vi "SPI读写.vi"(1 "DELAY":dbl, 3 "error in (no error)":errorcluster caption="错误输入（无错误）", 4 "从芯片读数据":string="spi r 0x04 0x0001", 5 "往芯片写数据":string="spi w 0x04 0x0001 0x01", 6 "VISA resource name":refnum<visa-resource-name>="COM3") -> (0 "error out":errorcluster, 2 "read buffer":string="spi read data is : 0xFF.")   [LabVIEW 2015]
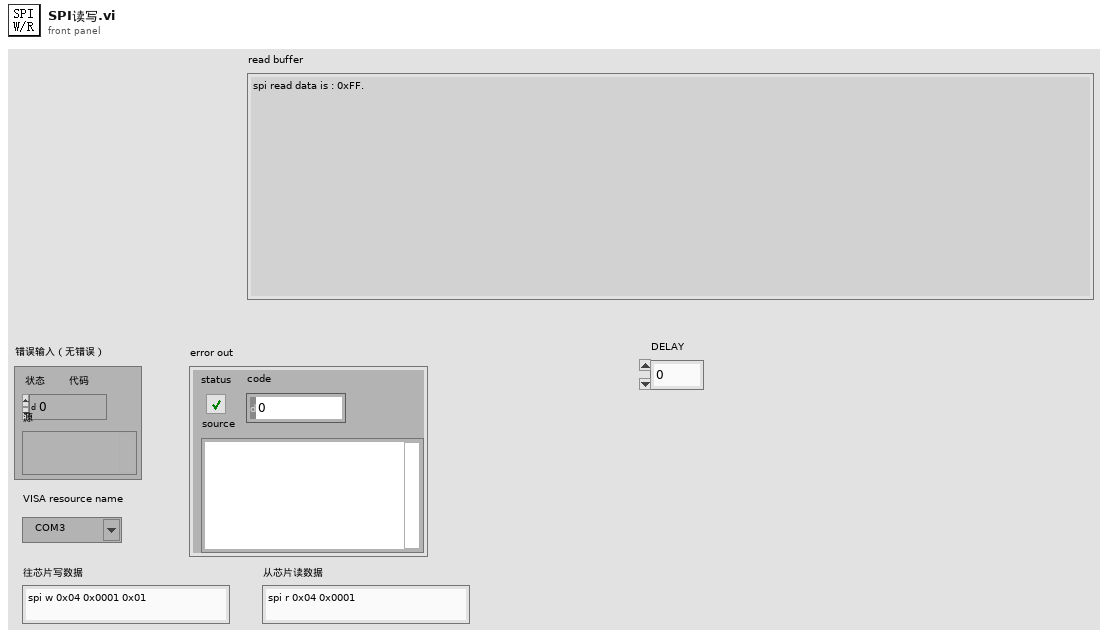
[diagram p1: front panel]
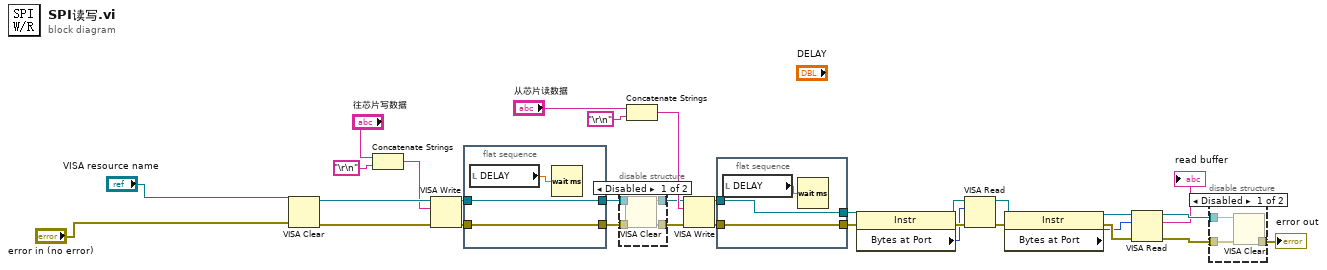
[diagram p0: block diagram]
diagram:
  n1 = VISA Clear(VISA resource name="VISA resource name", error in (no error)="error in (no error)") -> (VISA resource name out=w6:refnum<visa-resource-name>, error out=w7:errorcluster)
  n2 = Concatenate Strings("往芯片写数据", "\r\n") -> (w5:string)
  n3 = VISA Write(VISA resource name=w6, write buffer=w5, error in (no error)=w7) -> (VISA resource name out=w18:refnum<visa-resource-name>, error out=w17:errorcluster)  [unwired: 1 out]
  n4 = flat-sequence {
    tunnel: [w35] -> w13
    tunnel: w18 -> [w35]
    tunnel: [w34] -> w12
    tunnel: w17 -> [w34]
    frame #0 {
      n5 = local read "DELAY"() -> (w33:dbl)
      n6 = Wait (ms)(milliseconds to wait=w33) -> ()  [unwired: 1 out]
    }
  }
  n7 = disable-structure shown="Disabled" {
    disable-tunnel: w13 -> [w39 w41]
    disable-tunnel: w12 -> [w38 w40]
    disable-tunnel: [w37 w41] -> w11
    disable-tunnel: [w36 w40] -> w4
    frame Disabled {
      n8 = VISA Clear(VISA resource name=w39, error in (no error)=w38) -> (VISA resource name out=w37:refnum<visa-resource-name>, error out=w36:errorcluster)
    }
    frame Enabled {
    }
  }
  n9 = Concatenate Strings("从芯片读数据", "\r\n") -> (w14:string)
  n10 = VISA Write(VISA resource name=w11, write buffer=w14, error in (no error)=w4) -> (VISA resource name out=w22:refnum<visa-resource-name>, error out=w21:errorcluster)  [unwired: 1 out]
  n11 = flat-sequence {
    tunnel: [w44] -> w32
    tunnel: w22 -> [w44]
    tunnel: [w43] -> w30
    tunnel: w21 -> [w43]
    frame #0 {
      n12 = local read "DELAY"() -> (w42:dbl)
      n13 = Wait (ms)(milliseconds to wait=w42) -> ()  [unwired: 1 out]
    }
  }
  n14 = property class="Instr"(reference=w32, error in=w30) -> (reference out=w31:refnum<visa-resource-name>, error out=w29:errorcluster, "Bytes at Port"=w24:u32)
  n15 = VISA Read(VISA resource name=w31, byte count=w24, error in (no error)=w29) -> (VISA resource name out=w26:refnum<visa-resource-name>, error out=w25:errorcluster)  [unwired: 2 out]
  n16 = property class="Instr"(reference=w26, error in=w25) -> (reference out=w28:refnum<visa-resource-name>, error out=w27:errorcluster, "Bytes at Port"=w23:u32)
  n17 = VISA Read(VISA resource name=w28, byte count=w23, error in (no error)=w27) -> (VISA resource name out=w10:refnum<visa-resource-name>, read buffer=→"read buffer":string, error out=w8:errorcluster)  [unwired: 1 out]
  n18 = disable-structure shown="Disabled" {
    disable-tunnel: w10 -> [w47 _]
    disable-tunnel: [w46 w48] -> w9
    disable-tunnel: w8 -> [w45 w48]
    frame Disabled {
      n19 = VISA Clear(VISA resource name=w47, error in (no error)=w45) -> (error out=w46:errorcluster)  [unwired: 1 out]
    }
    frame Enabled {
    }
  }
  "error out" <- w9
